vi "yolo-detect.vi"() -> ()   [LabVIEW 2017]
uses:
  <vilib>/httpClient/POSTBuffer.vi
  <vilib>/wsapi/NI_WebServices.lvlib
  <vilib>/httpClient/LabVIEWHTTPClient.lvlib
panel:
  out "body":string="{\"result\":\"ok\",\"objects\":\"handbag - obj_id = 26,  x = 649, y = 239, w = 41, h = 79, prob = 0.901\\nhandbag - obj_id = 26,  x = 696, y = 328, w = 32, h = 63, prob = 0.529\\nbackpack - obj_id = 24,  x = 378, y = 288, w = 47, h = 34, prob = 0.743\\nhandbag - obj_id = 26,  x = 534, y = 228, w = 51, h = 146, prob = 0.278\\nhandbag - obj_id = 26,  x = 715, y = 324, w = 30, h = 37, prob = 0.261\\nhandbag - obj_id = 26,  x = 520, y = 291, w = 16, h = 30, prob = 0.234\\nhandbag - obj_id = 26,  x = 322, y = 230, w = 67, h = 142, prob = 0.217\\nperson - obj_id = 0,  x = 260, y = 198, w = 43, h = 115, prob = 0.614\\nperson - obj_id = 0,  x = 523, y = 194, w = 44, h = 83, prob = 0.546\\nperson - obj_id = 0,  x = 568, y = 210, w = 20, h = 50, prob = 0.478\\nperson - obj_id = 0,  x = 224, y = 207, w = 14, h = 50, prob = 0.472\\nperson - obj_id = 0,  x = 206, y = 205, w = 17, h = 50, prob = 0.457\\nperson - obj_id = 0,  x = 238, y = 209, w = 15, h = 46, prob = 0.448\\nperson - obj_id = 0,  x = 325, y = 210, w = 14, h = 45, prob = 0.415\\nperson - obj_id = 0,  x = 0, y = 201, w = 19, h = 69, prob = 0.406\\nperson - obj_id = 0,  x = 170, y = 207, w = 16, h = 22, prob = 0.289\\nperson - obj_id = 0,  x = 94, y = 206, w = 23, h = 19, prob = 0.283\\nperson - obj_id = 0,  x = 586, y = 209, w = 23, h = 40, prob = 0.278\\nperson - obj_id = 0,  x = 150, y = 206, w = 19, h = 18, prob = 0.268\\nperson - obj_id = 0,  x = 472, y = 234, w = 60, h = 145, prob = 0.99\\nbackpack - obj_id = 24,  x = 25, y = 198, w = 46, h = 53, prob = 0.728\\nperson - obj_id = 0,  x = 363, y = 199, w = 43, h = 78, prob = 0.867\\nbicycle - obj_id = 1,  x = 583, y = 246, w = 29, h = 66, prob = 0.404\\ncar - obj_id = 2,  x = 402, y = 225, w = 29, h = 46, prob = 0.248\\nperson - obj_id = 0,  x = 645, y = 196, w = 75, h = 203, prob = 0.969\\nperson - obj_id = 0,  x = 533, y = 234, w = 53, h = 146, prob = 0.971\\nbackpack - obj_id = 24,  x = 269, y = 207, w = 25, h = 34, prob = 0.718\\nperson - obj_id = 0,  x = 717, y = 198, w = 35, h = 111, prob = 0.813\\nperson - obj_id = 0,  x = 19, y = 177, w = 92, h = 167, prob = 0.979\\nbicycle - obj_id = 1,  x = 269, y = 254, w = 25, h = 67, prob = 0.902\\nbench - obj_id = 13,  x = 289, y = 282, w = 280, h = 96, prob = 0.581\\nbicycle - obj_id = 1,  x = 29, y = 255, w = 74, h = 128, prob = 0.923\\numbrella - obj_id = 25,  x = 465, y = 182, w = 62, h = 19, prob = 0.432\\nperson - obj_id = 0,  x = 118, y = 207, w = 12, h = 16, prob = 0.213\\nperson - obj_id = 0,  x = 318, y = 234, w = 76, h = 142, prob = 0.991\\ncar - obj_id = 2,  x = 82, y = 222, w = 142, h = 92, prob = 0.997\\n\"}"
  out "headers":string="HTTP/1.1 100 Continue\r\n\r\nHTTP/1.1 200 OK\r\nContent-Type: application/json\r\nContent-Length: 2573\r\nServer: Crow/0.2\r\nDate: Tue, 23 Feb 2021 06:51:12 GMT\r\n\r\n"
  in  "error in (no error)":errorcluster
  in  "yolo-server \"detect \"endpoint":string="http://localhost:18080/detect"
  out "string out (base64-encoded)":string="iVBORw0KGgoAAAANSUhEUgAAAwwAAAGQCAIAAACMJnA9AA5KZ0lEQVR4AQAGgPl/AO3q4e3q4e3r3+3r3+3r3+3r3+3r3u3r3vPx4nh2Z21sWoKBb2tqVnFwXHl4ZHNyYHNxZIB+cnx6bnZ0aHx5cHx5cH98dZCNhoqHgpyZlJGNipeTkM7Kye3p6Ojk4+jn4+bl4PP07MDAtmpqYG5sYMLAs+7o3NbQwJ+Wh52VgqqdjKuei7KjjpmKdY5+Z87BrsS+sn16cUJCOikqIh8gGiIlHiMmHxcaERQUDDc1KV5YTJ6VhrWol6WWgbKgirKgiLSeibmkj7ahjq2ciLSjk7msnKeZjId9cauimaqmnXVya2ZnYWBgXmlraIaKiVZVUTAmHDgoGT8vIHNkUcu8p7ChirOli7Oli7SmjLyulL2ul7mqlbytmriomJeHemxeUZCJeYiGd1JTS0BHQEdSTn6JhVtgWSQkGC4mEzMkDUMvFLWhhsCwl4yBa353Z7CtnLGwnrK0n6+woKOnmJuhk5aglZCckoeUi36OhHaGfEZSSF9rX5mhltHZysTKvNTXxOHfyKWfhWtnTJGNcpOPdIF9..."
  out "Original image":picture
  in  "path to JPEG file":path=path "E:/UPWORK/darknet/labview-meet-yolo/samples/001.png"
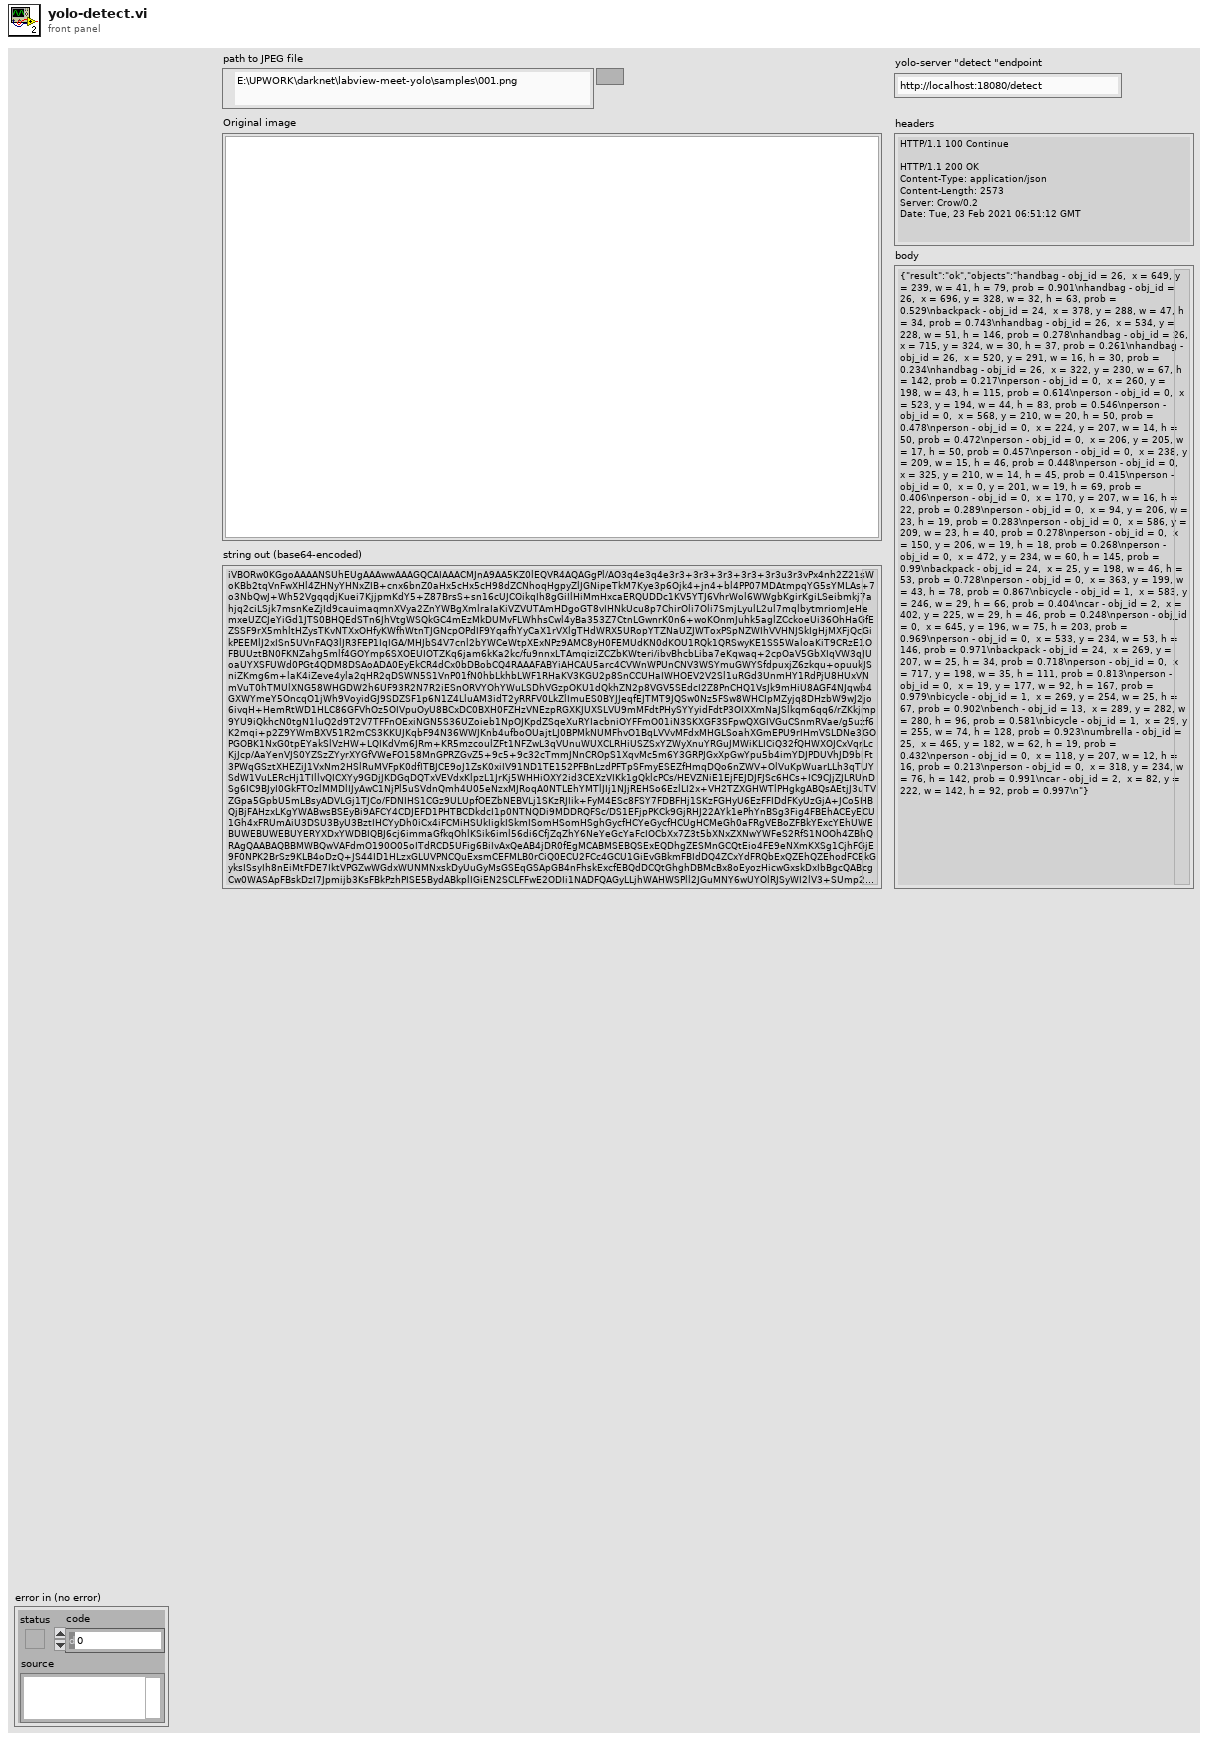
[diagram p1: front panel]
types:
  T1 = typedef "imagedata.ctl" = cluster{"image type":i32, "image depth":i32, "image":u8[], "mask":u8[], "colors":u32[], "Rectangle":cluster{"left":i16, "top":i16, "right":i16, "bottom":i16}}
  T2 = typedef "LabVIEWHTTPClient.lvlib/ClientHandle.ctl" = refnum<k1>
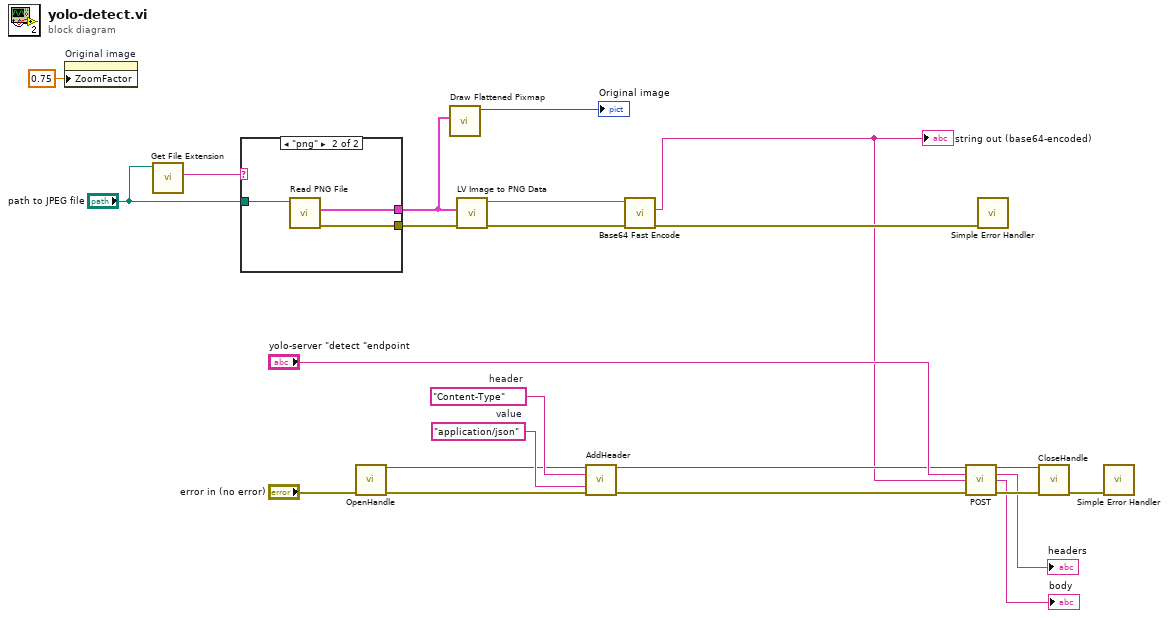
[diagram p0: block diagram]
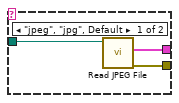
[diagram p2: hidden frame]
diagram:
  w17 = "application/json"  # value
  w16 = "Content-Type"  # header
  n1 = property on="Original image" class="Pict"("ZoomFactor"=sgl 0.75 ("Zoom Factor")) -> ()  [unwired: 2 in, 2 out]
  n2 = call <vilib>:"Get File Extension.vi"("file"="path to JPEG file") -> ("lowercase file extension"=w3:string)  [unwired: 6 in, 4 out]
  n3 = case shown="\"png\"" w3 {
    tunnel: [w25 w29] -> w23
    tunnel: [w24 w28] -> w21
    tunnel: "path to JPEG file" -> [w26 w27]
    frame "jpeg", "jpg", Default {
      n4 = call <vilib>:"Read JPEG File.vi"("path to JPEG file"=w26) -> ("error out"=w25:errorcluster, "image data"=w24:T1)  [unwired: 8 in, 1 out]
    }
    frame "png" {
      n5 = call <vilib>:"Read PNG File.vi"("path to PNG file"=w27) -> ("error out"=w29:errorcluster, "image data"=w28:T1)  [unwired: 8 in, 1 out]
    }
  }
  n6 = call <vilib>:"OpenHandle.vi"("error in (no error)"="error in (no error)") -> ("client handle out"=w10:T2, "error out"=w11:errorcluster)  [unwired: 13 in]
  n7 = call <vilib>:"Draw Flattened Pixmap.vi"("image data"=w21) -> ("new picture"=→"Original image":picture)  [unwired: 8 in]
  n8 = call <vilib>:"LV Image to PNG Data.vi"("error in (no error)"=w23, "image data"=w21) -> ("error out"=w19:errorcluster, "png data"=w20:string)  [unwired: 8 in]
  n9 = call <vilib>:"AddHeader.vi"("client handle"=w10, "header"=w16, "value"=w17, "error in (no error)"=w11) -> ("client handle out"=w7:T2, "error out"=w6:errorcluster)  [unwired: 10 in]
  n10 = call "Base64 Fast Encode.vi"("error in (no error)"=w19, "string in (not encoded)"=w20) -> ("error out"=w18:errorcluster, "string out (base64-encoded)"=w4:string)  [unwired: 8 in]
  "string out (base64-encoded)" <- w4
  n11 = call-poly <vilib>:"POST.vi"("client handle"=w7, "url"="yolo-server \"detect \"endpoint", "buffer"=w4, "error in (no error)"=w6) -> ("client handle out"=w12:T2, "headers"=→"headers":string, "body"=→"body":string, "error out"=w13:errorcluster)  [unwired: 8 in]
  n12 = call <vilib>:"Simple Error Handler.vi"("error in (no error)"=w18) -> ()  [unwired: 4 in, 5 out]
  n13 = call <vilib>:"CloseHandle.vi"("client handle"=w12, "error in (no error)"=w13) -> ("error out"=w5:errorcluster)  [unwired: 13 in]
  n14 = call <vilib>:"Simple Error Handler.vi"("error in (no error)"=w5) -> ()  [unwired: 4 in, 5 out]
